vi "Estimate Differential Steering Frame.vi"(8 "error in (no error)":errorcluster, 11 "steering frame in":refnum<class "NI_Robotics_Steering Frame.lvclass">) -> (0 "error out":errorcluster, 2 "estimated differential steering frame copy":refnum<class "NI_Robotics_Differential Steering Frame.lvclass">, 3 "steering frame out":refnum<class "NI_Robotics_Steering Frame.lvclass">)   [LabVIEW 2017, in "NI_Robotics_Configure Steering Frame.lvlib"]
uses:
  <vilib>/robotics/Dialog/Configure Steering Frame/NI_Robotics_Configure Steering Frame.lvlib
  <vilib>/robotics/Steering/Steering Frame/NI_Robotics_Steering Frame.lvclass
  <vilib>/robotics/Steering/Differential Steering Frame/NI_Robotics_Differential Steering Frame.lvclass
  <vilib>/robotics/Steering/Steering Frame/NI_Robotics_Steering Frame.lvclass/NI_Robotics_Steering Frame.ctl
  <vilib>/robotics/Steering/Wheel/Wheel Parameters.ctl
  <vilib>/robotics/Steering/Wheel/Rotation Direction.ctl
  <vilib>/robotics/Steering/Fixed Wheel/NI_Robotics_Fixed Wheel.lvclass
  c:/Program Files (x86)/National Instruments/LabVIEW 2017/vi.lib/robotics/Steering/Wheel/NI_Robotics_Wheel.lvclass
  <vilib>/robotics/Steering/Wheel/NI_Robotics_Wheel.lvclass/NI_Robotics_Wheel.ctl
  <vilib>/robotics/Steering/Steering Frame/Get Multiple Wheels in Steering Frame.vi
  <vilib>/robotics/Steering/Wheel/Get General Wheel Information.vi
  <vilib>/robotics/Steering/Wheel/Get Wheel Radius.vi
  <vilib>/robotics/Steering/Wheel/Get Motor Communication.vi
  <vilib>/robotics/Steering/Wheel/Get Wheel Parameters.vi
  <vilib>/robotics/Steering/Differential Steering Frame/Create Differential Steering Frame.vi
  <vilib>/robotics/Steering/Omnidirectional Wheel/Create Omnidirectional Wheel.vi
  <vilib>/robotics/Steering/Mecanum Wheel/Create Mecanum Wheel.vi
  <vilib>/robotics/Steering/Caster Wheel/Create Caster Wheel.vi
  <vilib>/robotics/Steering/Steering Wheel/Create Steering Wheel.vi
  <vilib>/robotics/Steering/Fixed Wheel/Create Fixed Wheel.vi
  <vilib>/robotics/Steering/Wheel/NI_Robotics_Wheel.lvclass
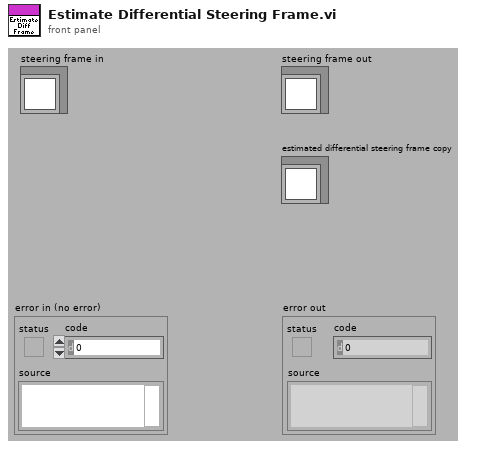
[diagram p1: front panel]
types:
  T1 = typedef "NI_Robotics_Wheel.lvclass/Wheel Parameters.ctl" = cluster{"wheel radius":dbl, "gear ratio":dbl, "forward rotation direction":T2}
  T2 = typedef "NI_Robotics_Wheel.lvclass/Rotation Direction.ctl" = u16
  T3 = cluster{"[0]":refnum<class "NI_Robotics_Fixed Wheel.lvclass">, "[1]":refnum<class "NI_Robotics_Fixed Wheel.lvclass">}
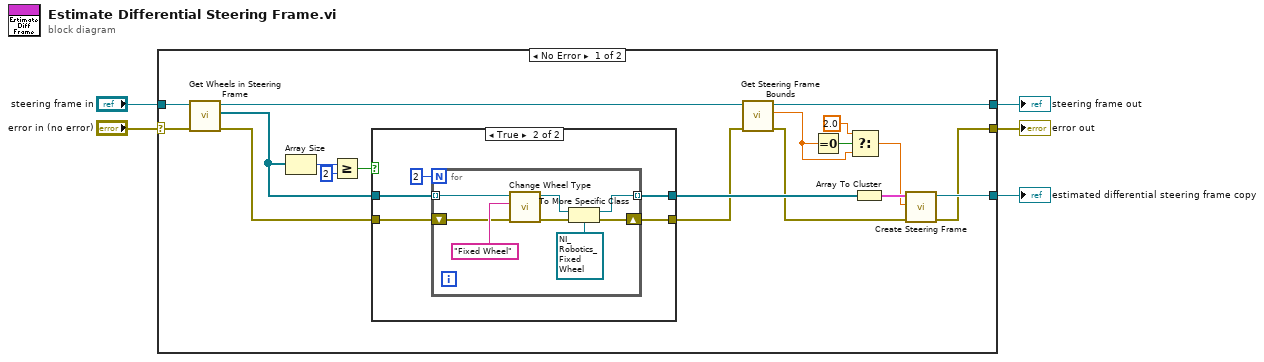
[diagram p0: block diagram]
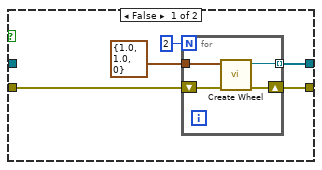
[diagram p2: hidden frame]
diagram:
  n1 = case shown="No Error" "error in (no error)" {
    selector: "error in (no error)" -> [w24 w48]
    tunnel: [w21 w48] -> w4
    tunnel: "steering frame in" -> [w23 w47]
    tunnel: [w13 w47] -> w2
    tunnel: [w22 _] -> w1
    frame No Error {
      n2 = call-poly <vilib>:"Get Wheels in Steering Frame.vi"("error in (no error)"=w24, "steering frame in"=w23) -> ("error out"=w16:errorcluster, "wheels"=w17:refnum<class "NI_Robotics_Wheel.lvclass">[], "steering frame out"=w6:refnum<class "NI_Robotics_Steering Frame.lvclass">)  [unwired: 3 in, 4 out]
      n3 = Array Size(array=w17) -> (size(s)=w20:i32)
      n4 = Greater Or Equal?(x=w20, y=2) -> (x >= y?=w18:bool)
      n5 = case shown="True" w18 {
        tunnel: w17 -> [_ w37]
        tunnel: w16 -> [w27 w34]
        tunnel: [w26 w35] -> w15
        tunnel: [w25 w36] -> w7
        frame False {
          n6 = for {
            N: 2 -> [_]
            tunnel: T1 {"wheel radius"=1.0, "gear ratio"=1.0, "forward rotation direction"=0} ("wheel parameters") -> [w33]
            shift-right: [w31] -> w25
            shift-left: w27 -> [w32]
            tunnel: [w30] -> w26 mode=indexing
            n7 = call-poly <vilib>:"Create Wheel.vi"("error in (no error)"=w32, "wheel parameters"=w33) -> ("error out"=w31:errorcluster, "fixed wheel out"=w30:refnum<class "NI_Robotics_Fixed Wheel.lvclass">)  [unwired: 8 in]
          }
        }
        frame True {
          n8 = for {
            N: 2 -> [_]
            tunnel: w37 -> [w46] mode=indexing
            shift-right: [w42] -> w36
            shift-left: w34 -> [w44]
            tunnel: [w40] -> w35 mode=indexing
            n9 = call <vilib>:"Change Wheel Type.vi"("error in (no error)"=w44, "wheel type"="Fixed Wheel", "wheel in"=w46) -> ("error out"=w43:errorcluster, "wheel out"=w41:refnum<class "NI_Robotics_Wheel.lvclass">)  [unwired: 6 in, 1 out]
            n10 = To More Specific Class(target class=refnum<class "NI_Robotics_Fixed Wheel.lvclass"> refnum ("fixed wheel out"), reference=w41, error in=w43) -> (specific class reference=w40:refnum<class "NI_Robotics_Fixed Wheel.lvclass">, error out=w42:errorcluster)
          }
        }
      }
      n11 = call <vilib>:"Get Steering Frame Bounds.vi"("error in (no error)"=w7, "steering frame in"=w6) -> ("error out"=w8:errorcluster, "width"=w11:dbl, "steering frame out"=w13:refnum<class "NI_Robotics_Steering Frame.lvclass">)  [unwired: 4 in, 3 out]
      n12 = Equal To 0?(x=w11) -> (x = 0?=w12:bool)
      n13 = Select(t=2.0 ("wheel separation"), s=w12, f=w11) -> (s? t:f=w9:dbl)
      n14 = Array To Cluster(array=w15) -> (cluster=w14:T3)
      n15 = call-poly <vilib>:"Create Steering Frame.vi"("error in (no error)"=w8, "wheel separation"=w9, "wheels"=w14) -> ("error out"=w21:errorcluster, "differential steering frame out"=w22:refnum<class "NI_Robotics_Differential Steering Frame.lvclass">)  [unwired: 7 in]
    }
    frame Error {
    }
  }
  "steering frame out" <- w2
  "error out" <- w4
  "estimated differential steering frame copy" <- w1
